vi "Ctor.vi"(6 "This VI":refnum<vi>, 8 "error in (no error)":errorcluster) -> (0 "error out":errorcluster, 3 "Application out":refnum<class "Application.lvclass">)   [LabVIEW 2024, in "Application.lvclass"]
uses:
  Application.lvclass
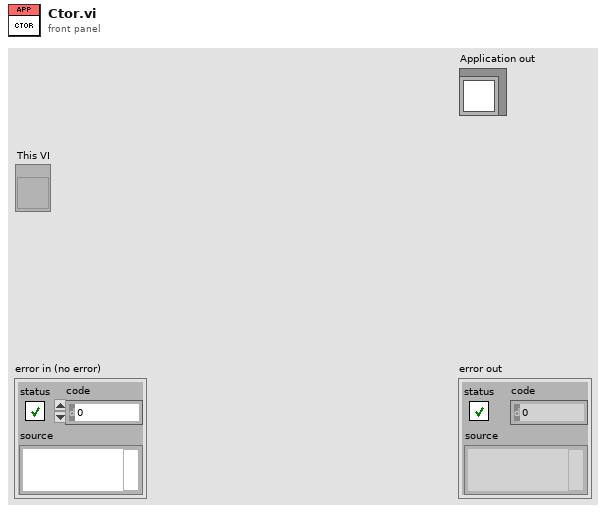
[diagram p1: front panel]
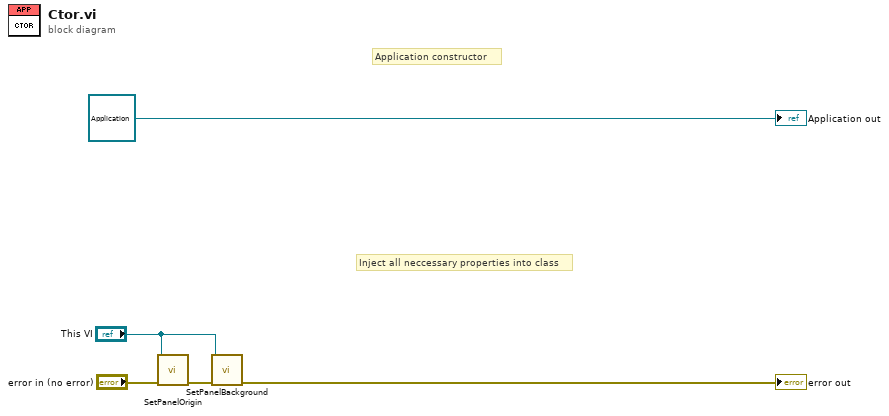
[diagram p0: block diagram]
diagram:
  # "Inject all neccessary properties into class"
  # "Application constructor"
  n1 = call "SetPanelOrigin.vi"("error in (no error)"="error in (no error)", "VI in"="This VI") -> ("error out"=w4:errorcluster)  [unwired: 9 in]
  n2 = call "SetPanelBackground.vi"("error in (no error)"=w4, "VI in"="This VI") -> ("error out"=→"error out":errorcluster)  [unwired: 9 in]
  "Application out" <- refnum<class "Application.lvclass"> refnum ("Application in")
